vi "Set Current Dye Values.vi"(8 "error in (no error)":errorcluster, 9 "Dye Settings":T1={"Dye Name"="", "Pulse Sequence"=[], "Emission Filter"=0, "Exposure (s)"=0.01, "Yellow Select"=FALSE, "# Pulses"=1} {"# Pulses" min=1 max=100; "Exposure (s)" min=1.0 max=5000.0}, 10 "index":i32, 11 "Settings in":refnum<class "Settings.lvclass">) -> (0 "error out":errorcluster, 3 "Settings out":refnum<class "Settings.lvclass">)   [LabVIEW 2010, in "Settings.lvclass"]
uses:
  Settings.lvclass
  Settings.lvclass/Settings.ctl
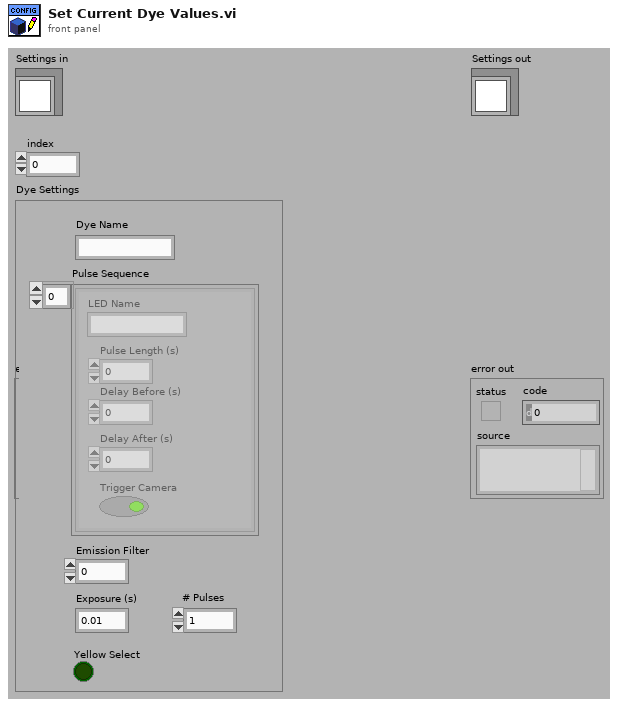
[diagram p1: front panel]
types:
  T1 = cluster{"Dye Name":string, "Pulse Sequence":cluster{"LED Name":string, "Pulse Length (s)":dbl, "Delay Before (s)":dbl, "Delay After (s)":dbl, "Trigger Camera":bool}[], "Emission Filter":i16, "Exposure (s)":dbl, "Yellow Select":bool, "# Pulses":i32}
  T2 = cluster{"Dye Name":string, "Pulse Sequence":cluster{"LED Name":string, "Pulse Length (s)":dbl, "Delay Before (s)":dbl, "Delay After (s)":dbl, "Trigger Camera":bool}[], "Emission Filter":i16, "Exposure (s)":dbl, "Yellow Select":bool, "# Pulses":i32}[]
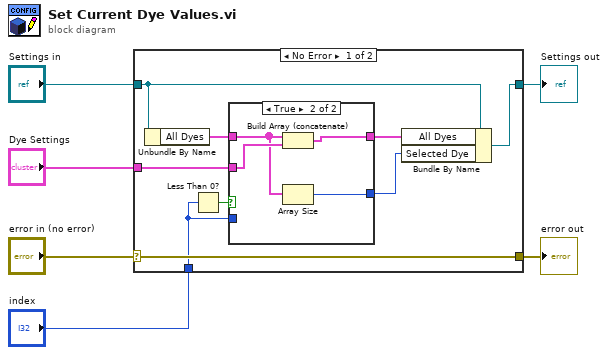
[diagram p0: block diagram]
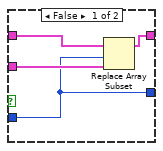
[diagram p2: hidden frame]
diagram:
  n1 = case shown="No Error" "error in (no error)" {
    selector: "error in (no error)" -> [w15 w24]
    tunnel: [w15 w24] -> w5
    tunnel: [w14 w25] -> w3
    tunnel: "Settings in" -> [w13 w25]
    tunnel: "Dye Settings" -> [w10 _]
    tunnel: "index" -> [w9 _]
    frame No Error {
      n2 = Unbundle By Name(w13) -> ("All Dyes"=w12:T2)
      n3 = Less Than 0?(x=w9) -> (x < 0?=w8:bool)
      n4 = case shown="True" w8 {
        tunnel: w12 -> [w19 w21]
        tunnel: [w18 w23] -> w11
        tunnel: w10 -> [w17 w22]
        tunnel: w9 -> [w16 _]
        tunnel: [w16 w20] -> w7
        frame False {
          n5 = Replace Array Subset(array=w19, new element=w17, index=w16) -> (w18:T2)
        }
        frame True {
          n6 = Build Array (concatenate)(w21, w22) -> (w23:T2)
          n7 = Array Size(array=w21) -> (size(s)=w20:i32)
        }
      }
      n8 = Bundle By Name(cluster=w13, "All Dyes"=w11, "Selected Dye"=w7) -> (w14:refnum<class "Settings.lvclass">)
    }
    frame Error {
    }
  }
  "error out" <- w5
  "Settings out" <- w3
